vi "Configure Trigger (Edge).vi"(0 "VISA resource name":refnum<visa-resource-name>, 1 "Trigger Coupling (0 : DC)":u16(ring) items=["DC", "HF Reject", "LF Reject", "Noise Reject", "AC"], 5 "Trigger Source (0: Channel 1)":u16(ring) items=["Channel 1", "Channel 2", "Channel 3", "Channel 4", "AC Line", "Aux", "Digital Channel 0", "Digital Channel 1", "Digital Channel 2", "Digital Channel 3", "Digital Channel 4", "Digital Channel 5", "Digital Channel 6", "Digital Channel 7", "Digital Channel 8", "Digital Channel 9", "Digital Channel 10", "Digital Channel 11", "Digital Channel 12", "Digital Channel 13", "Digital Channel 14", "Digital Channel 15", "RF"], 7 "Trigger Level (0.0 V)":dbl, 9 "Trigger Slope (0: Rising)":u16(ring) items=["Rising", "Falling"], 11 "error in (no error)":errorcluster) -> (4 "VISA resource name out":refnum<visa-resource-name>, 15 "error out":errorcluster)   [LabVIEW 2009, in "Tektronix DPO MSO 2000 4000 Series.lvlib"]
doc: "Configures edge trigger settings for an oscilloscope. An edge trigger occurs when the trigger signal passes through the voltage threshold that you specify in <B>Trigger Level</B> and has the slope that you specify in <B>Trigger Slope</B>."
uses:
  <instrlib>/Tektronix DPO MSO 2000 4000 Series/Tektronix DPO MSO 2000 4000 Series.lvlib
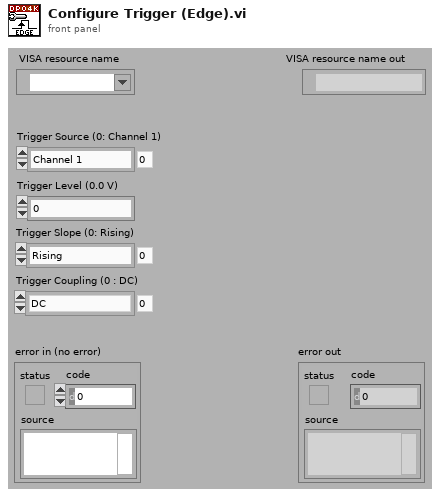
[diagram p1: front panel]
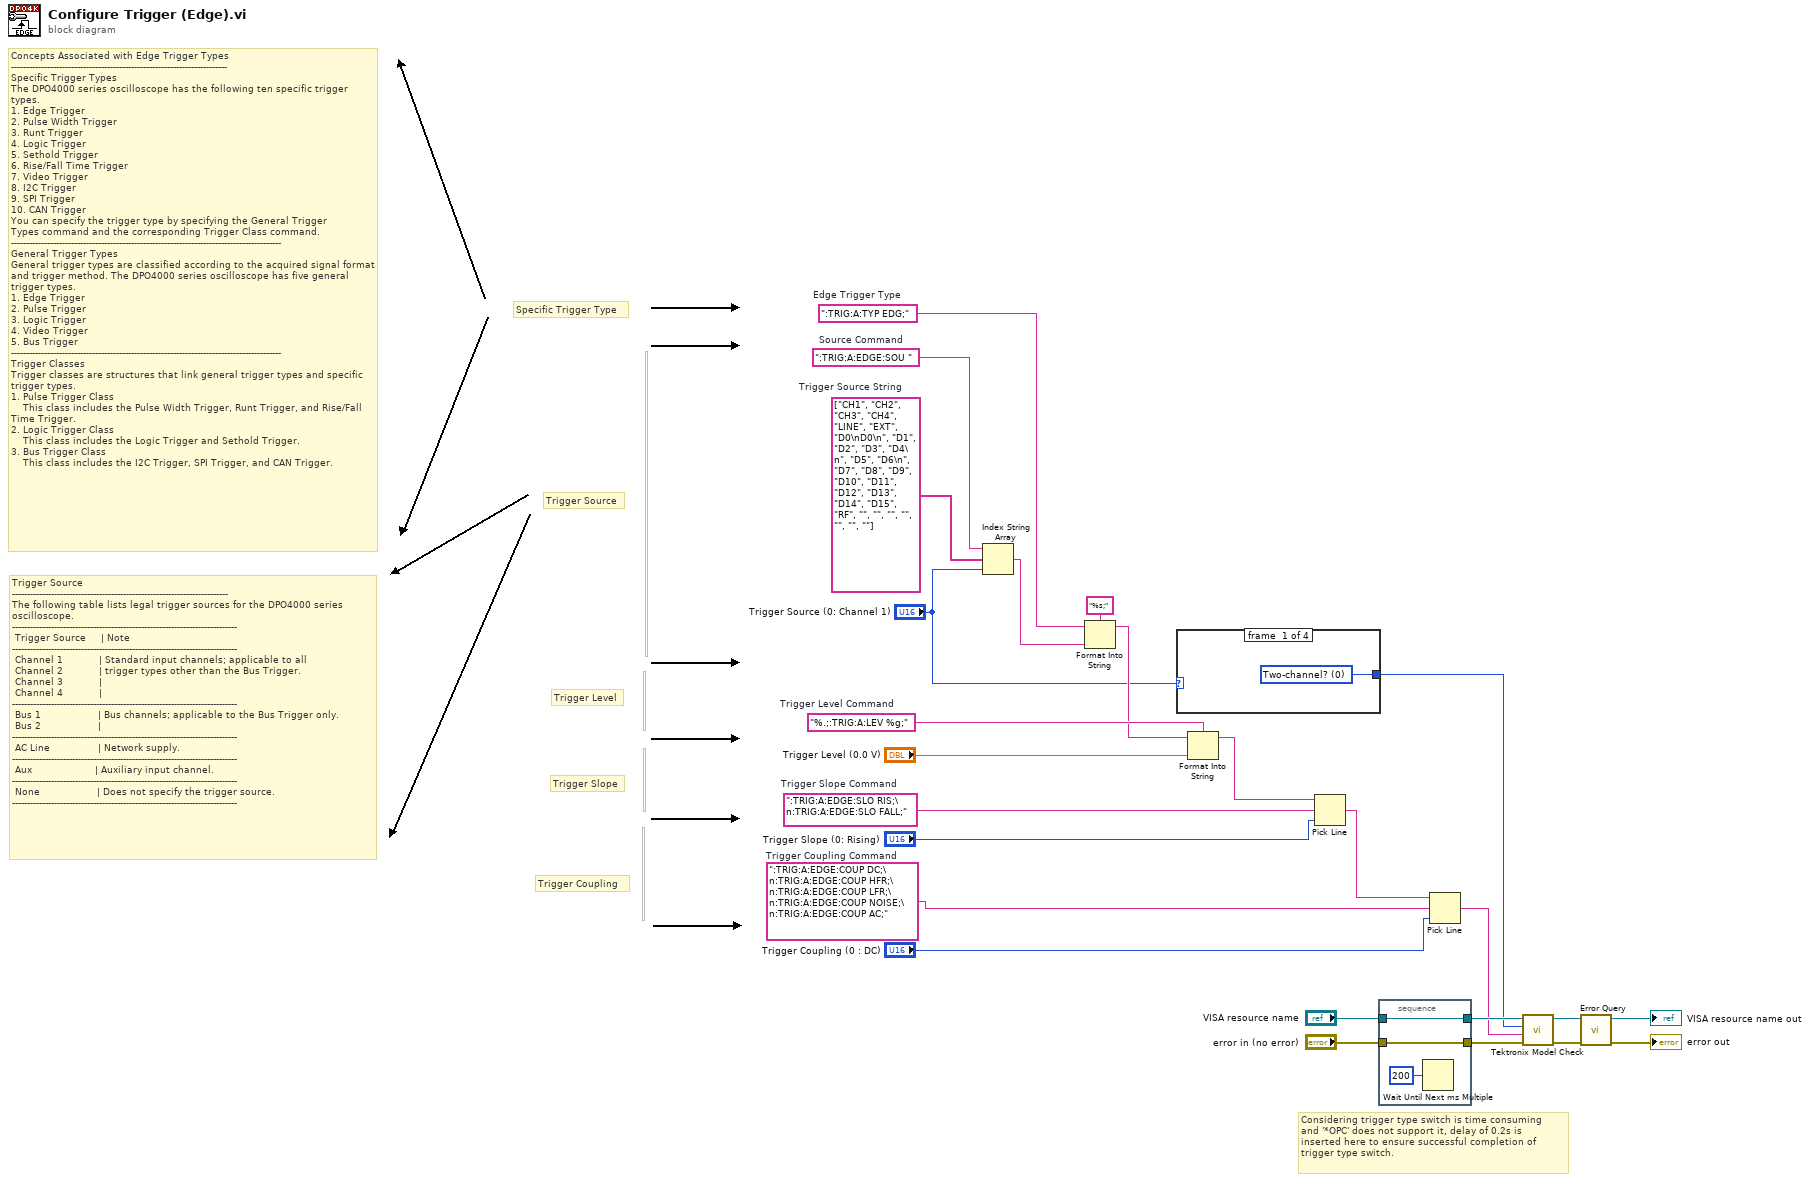
[diagram p0: block diagram]
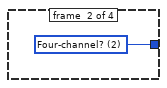
[diagram p2: hidden frame]
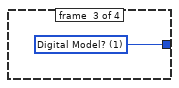
[diagram p3: hidden frame]
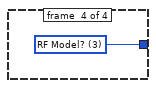
[diagram p4: hidden frame]
diagram:
  w13 = ":TRIG:A:EDGE:COUP DC;\n:TRIG:A:EDGE:COUP HFR;\n:TRIG:A:EDGE:COUP LFR;\n:TRIG:A:EDGE:COUP NOISE;\n:TRIG:A:EDGE:COUP AC;"  # Trigger Coupling Command
  w19 = string[] ["CH1", "CH2", "CH3", "CH4", "LINE", "EXT", "D0\nD0\n", "D1", "D2", "D3", "D4\n", "D5", "D6\n", "D7", "D8", "D9", "D10", "D11", "D12", "D13", "D14", "D15", "RF", "", "", "", "", "", "", ""]  # Trigger Source String
  w21 = ":TRIG:A:EDGE:SLO RIS;\n:TRIG:A:EDGE:SLO FALL;"  # Trigger Slope Command
  w23 = "%.;:TRIG:A:LEV %g;"  # Trigger Level Command
  w17 = ":TRIG:A:TYP EDG;"  # Edge Trigger Type
  w18 = ":TRIG:A:EDGE:SOU "  # Source Command
  # "Trigger Source\n------------------------------------------------------------------------\nThe following table lists legal trigger sources for the DPO4000 series oscilloscope.\n---------------------------------------------------------------------------\n Trigger Source     | Note                                                           \n---------------------------------------------------------------------------\n Channel 1            | Standard input channels; applicable to all      \n Channel 2            | trigger types other than the Bus Trigger.         \n Channel 3            |     \n Channel 4            |\n---------------------------------------------------------------------------\n Bus 1                   | Bus channels; applicable to the Bus Trigger only.\n Bus 2                   | \n---------------------------------------------------------------------------\n AC Line                | Network supply.\n---------------------------------------------------------------------------\n Aux                     | Auxiliary input channel.\n---------------------------------------------------------------------------\n None                   | Does not specify the trigger source.\n---------------------------------------------------------------------------"
  # "Trigger Coupling"
  # "Trigger Slope"
  # "Trigger Level"
  # "Trigger Source"
  # "Specific Trigger Type"
  # "Concepts Associated with Edge Trigger Types\n------------------------------------------------------------------------\nSpecific Trigger Types\nThe DPO4000 series oscilloscope has the following ten specific trigger types.\n1. Edge Trigger\n2. Pulse Width Trigger\n3. Runt Trigger\n4. Logic Trigger\n5. Sethold Trigger\n6. Rise/Fall Time Trigger\n7. Video Trigger\n8. I2C Trigger\n9. SPI Trigger\n10. CAN Trigger\nYou can specify the trigger type by specifying the General Trigger \nTypes command and the corresponding Trigger Class command.\n------------------------------------------------------------------------------------------\nGeneral Trigger Types \nGeneral trigger types are classified according to the acquired signal format and trigger method. The DPO4000 series oscilloscope has five general trigger types.\n1. Edge Trigger\n2. Pulse Trigger\n3. Logic Trigger\n4. Video Trigger\n5. Bus Trigger\n------------------------------------------------------------------------------------------\nTrigger Classes\nTrigger classes are structures that link general trigger types and specific trigger types.\n1. Pulse Trigger Class\n    This class includes the Pulse Width Trigger, Runt Trigger, and Rise/Fall Time Trigger.\n2. Logic Trigger Class\n    This class includes the Logic Trigger and Sethold Trigger.\n3. Bus Trigger Class\n    This class includes the I2C Trigger, SPI Trigger, and CAN Trigger."
  # "Considering trigger type switch is time consuming\nand '*OPC' does not support it, delay of 0.2s is \ninserted here to ensure successful completion of\ntrigger type switch."
  n1 = Index String Array(1:"Trigger Source (0: Channel 1)", 2:w19, 3:w18) -> (0:w15:string)
  n2 = Format Into String(format string="%s;", initial string=w17, w15) -> (resulting string=w14:string)  [unwired: 1 in, 1 out]
  n3 = case shown="0, 1, 4, 5, Default" "Trigger Source (0: Channel 1)" {
    tunnel: [w26 w27 w28 w29] -> w1
    frame #0 {
      w26 = u16 0 items=["Two-channel?", "Digital Model?", "Four-channel?", "RF Model?"] ("Oscilloscope Model Tests (3: RF Model?)")
    }
    frame #1 {
      w27 = u16 2 items=["Two-channel?", "Digital Model?", "Four-channel?", "RF Model?"] ("Oscilloscope Model Tests (3: RF Model?)")
    }
    frame #2 {
      w28 = u16 1 items=["Two-channel?", "Digital Model?", "Four-channel?", "RF Model?"] ("Oscilloscope Model Tests (3: RF Model?)")
    }
    frame #3 {
      w29 = u16 3 items=["Two-channel?", "Digital Model?", "Four-channel?", "RF Model?"] ("Oscilloscope Model Tests (3: RF Model?)")
    }
  }
  n4 = Format Into String(format string=w23, initial string=w14, "Trigger Level (0.0 V)") -> (resulting string=w11:string)  [unwired: 1 in, 1 out]
  n5 = Pick Line(string ("")=w11, multi-line string=w21, line index="Trigger Slope (0: Rising)") -> (output string=w10:string)
  n6 = stacked-sequence {
    tunnel: "VISA resource name" -> [w31]
    tunnel: [w31] -> w7
    tunnel: "error in (no error)" -> [w30]
    tunnel: [w30] -> w6
    frame #0 {
      n7 = Wait Until Next ms Multiple(millisecond multiple=u32 200) -> ()  [unwired: 1 out]
    }
  }
  n8 = Pick Line(string ("")=w10, multi-line string=w13, line index="Trigger Coupling (0 : DC)") -> (output string=w3:string)
  n9 = call <instrlib>:"Tektronix Model Check.vi"("error in (no error)"=w6, "Command String"=w3, "Oscilloscope Model Tests (3: RF Model?)"=w1, "VISA resource name"=w7) -> ("error out"=w4:errorcluster, "VISA resource name out"=w5:refnum<visa-resource-name>)  [unwired: 6 in]
  n10 = call <instrlib>:"Error Query.vi"("error in (no error)"=w4, "VISA resource name"=w5) -> ("error out"=→"error out":errorcluster, "VISA resource name out"=→"VISA resource name out":refnum<visa-resource-name>)  [unwired: 6 in, 2 out]
